vi "File_Size Folder to Max Files.vi"(8 "Error":errorcluster, 9 "Max Size":i32, 11 "Folder":path) -> (0 "Error Out":errorcluster, 3 "Removed Count Out":i32)   [LabVIEW 2020]
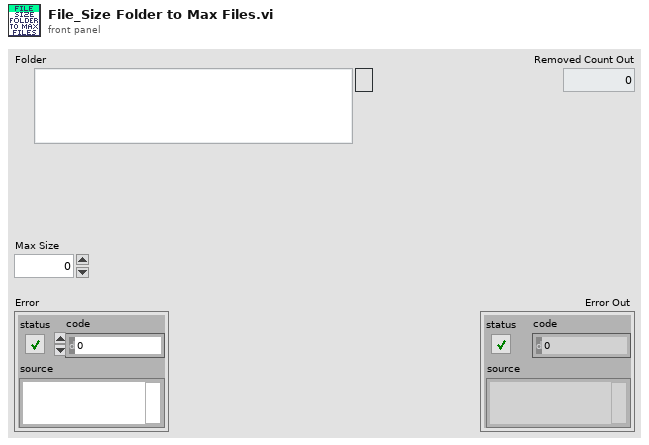
[diagram p1: front panel]
types:
  T1 = cluster{"last mod":timestamp, "appended path":path}
  T2 = cluster{"last mod":timestamp, "appended path":path}[]
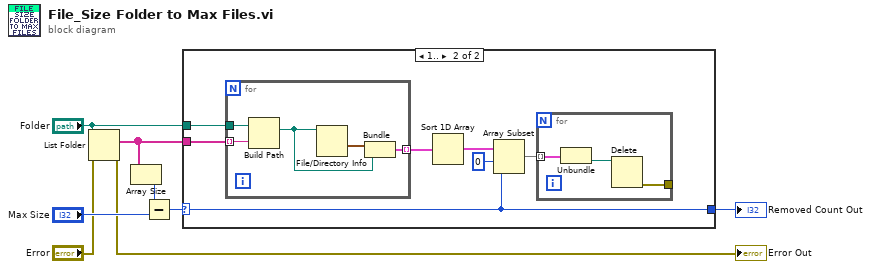
[diagram p0: block diagram]
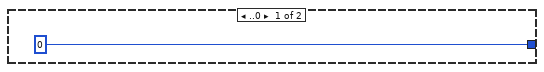
[diagram p2: hidden frame]
diagram:
  n1 = List Folder(path="Folder", error in="Error") -> (filenames=w7:string[], error out=→"Error Out":errorcluster)  [unwired: 2 in, 2 out]
  n2 = Array Size(array=w7) -> (size(s)=w6:i32)
  n3 = Subtract(x=w6, y="Max Size") -> (x-y=w4:i32)
  n4 = case shown="1.." w4 {
    selector: w4 -> [_ w10]
    tunnel: "Folder" -> [_ w16]
    tunnel: w7 -> [_ w14]
    tunnel: [0 w10] -> w1
    frame ..0 {
    }
    frame 1.. {
      n5 = for {
        tunnel: w14 -> [w24] mode=indexing
        tunnel: w16 -> [w23]
        tunnel: [w20] -> w15 mode=indexing
        n6 = Build Path(base path=w23, name or relative path=w24) -> (appended path=w21:path)
        n7 = File/Directory Info(path=w21) -> (last mod=w22:timestamp)  [unwired: 1 in, 6 out]
        n8 = Bundle("last mod"=w22, "appended path"=w21) -> (w20:T1)  [unwired: 1 in]
      }
      n9 = Sort 1D Array(array=w15) -> (sorted array=w13:T2)
      n10 = Array Subset(array=w13, index=0, length=w10) -> (w11:T2)
      n11 = for {
        tunnel: w11 -> [w19] mode=indexing
        tunnel: [w17] -> _
        n12 = Unbundle(w19) -> ("appended path"=w18:path)  [unwired: 1 out]
        n13 = Delete(path (use dialog)=w18) -> (error out=w17:errorcluster)  [unwired: 4 in, 2 out]
      }
    }
  }
  "Removed Count Out" <- w1
